vi "Get Config.vi"(8 "error in (no error)":errorcluster, 11 "DeploySerialResource in":refnum<class "SerialResource.lvclass">) -> (0 "error out":errorcluster, 2 "Config":T1[](array[typedef]), 3 "DeploySerialResource out":refnum<class "SerialResource.lvclass">)   [LabVIEW 2020, in "PicoG-Core.lvlib" / "SerialResource.lvclass"]
uses:
  SerialResource.lvclass
  SerialResource.lvclass/SerialResource.ctl
  Resource/Config Item.ctl
  Resource/Resource.lvclass
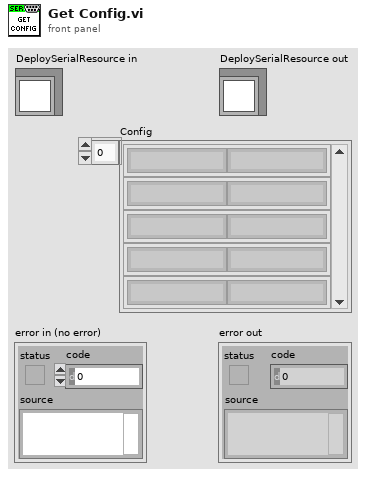
[diagram p1: front panel]
types:
  T1 = typedef "PicoG-Core.lvlib/Resource.lvclass/Config Item.ctl" = cluster{"Key":string, "Value":string}
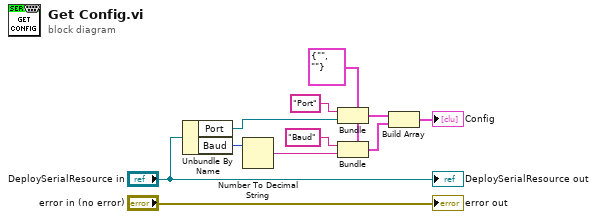
[diagram p0: block diagram]
diagram:
  w8 = T1 {"Key"="", "Value"=""} ("Config Item")
  n1 = Unbundle By Name("DeploySerialResource in") -> ("Port"=w5:refnum<visa-resource-name>, "Baud"=w9:u32)
  n2 = Number To Decimal String(number=w9) -> (decimal integer string=w7:string)  [unwired: 1 in]
  n3 = Bundle(cluster=w8, "Key"="Port", "Value"=w5) -> (w3:T1)
  n4 = Bundle(cluster=w8, "Key"="Baud", "Value"=w7) -> (w2:T1)
  n5 = Build Array(w3, w2) -> (→"Config":T1[])
  "error out" <- "error in (no error)"
  "DeploySerialResource out" <- "DeploySerialResource in"
